vi "TMCM351- setDecay.vi"(3 "错误输入":errorcluster caption="错误输入（无错误）", 5 "com in":refnum<visa-resource-name>) -> (0 "错误输出":errorcluster, 2 "com out":refnum<visa-resource-name>)   [LabVIEW 2018]
uses:
  module_param.vi
panel:
  # "203 \n衰减"
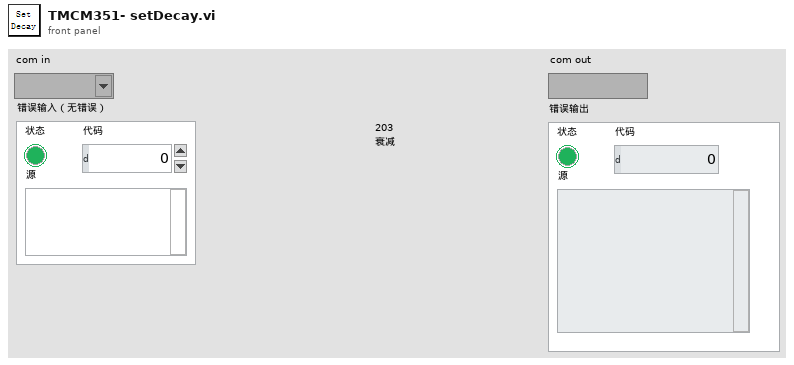
[diagram p1: front panel]
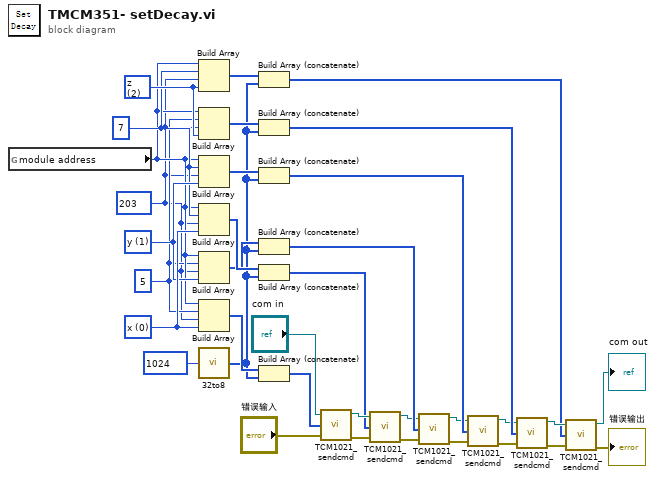
[diagram p0: block diagram]
diagram:
  w18 = u8 2 items=["x", "y", "z"] ("motor")
  w23 = u8 1 items=["x", "y", "z"] ("motor")
  w33 = u8 0 items=["x", "y", "z"] ("motor")
  w17 = u8 7 ("元素")
  w1 = u8 203
  w15 = u8 5
  n1 = global read "module_param.vi" "module address"() -> (w16:u8)
  n2 = Build Array(w16, w17, w1, w18) -> (w14:u8[])
  n3 = Build Array(w16, w15, w1, w18) -> (w13:u8[])
  n4 = Build Array(w16, w17, w1, w23) -> (w22:u8[])
  n5 = Build Array(w16, w17, w1, w33) -> (w32:u8[])
  n6 = Build Array(w16, w15, w1, w23) -> (w21:u8[])
  n7 = Build Array(w16, w15, w1, w33) -> (w35:u8[])
  n8 = call "32to8.vi"("32data_in"=1024 ("Acclation")) -> ("8Array"=w12:u8[])
  n9 = Build Array (concatenate)(w14, w12) -> (w10:u8[])
  n10 = Build Array (concatenate)(w13, w12) -> (w11:u8[])
  n11 = Build Array (concatenate)(w22, w12) -> (w19:u8[])
  n12 = Build Array (concatenate)(w21, w12) -> (w20:u8[])
  n13 = Build Array (concatenate)(w32, w12) -> (w26:u8[])
  n14 = Build Array (concatenate)(w35, w12) -> (w29:u8[])
  n15 = call "TCM1021_sendcmd.vi"("com in"="com in", "command in"=w29, "错误输入"="错误输入") -> ("com out"=w28:refnum<visa-resource-name>, "错误输出"=w27:errorcluster)  [unwired: 2 out]
  n16 = call "TCM1021_sendcmd.vi"("com in"=w28, "command in"=w26, "错误输入"=w27) -> ("com out"=w5:refnum<visa-resource-name>, "错误输出"=w4:errorcluster)  [unwired: 2 out]
  n17 = call "TCM1021_sendcmd.vi"("com in"=w5, "command in"=w20, "错误输入"=w4) -> ("com out"=w7:refnum<visa-resource-name>, "错误输出"=w6:errorcluster)  [unwired: 2 out]
  n18 = call "TCM1021_sendcmd.vi"("com in"=w7, "command in"=w19, "错误输入"=w6) -> ("com out"=w9:refnum<visa-resource-name>, "错误输出"=w8:errorcluster)  [unwired: 2 out]
  n19 = call "TCM1021_sendcmd.vi"("com in"=w9, "command in"=w11, "错误输入"=w8) -> ("com out"=w25:refnum<visa-resource-name>, "错误输出"=w24:errorcluster)  [unwired: 2 out]
  n20 = call "TCM1021_sendcmd.vi"("com in"=w25, "command in"=w10, "错误输入"=w24) -> ("com out"=→"com out":refnum<visa-resource-name>, "错误输出"=→"错误输出":errorcluster)  [unwired: 2 out]
